vi "PH_Stepmotor_BaseClass.update Axes Config GUI.vi"(0 "VI in":refnum<vi>, 5 "error in (no error)":errorcluster) -> (14 "VI out":refnum<vi>, 19 "error out":errorcluster)   [LabVIEW 2014, in "PH_Stepmotor_BaseClass.lvlib"]
doc: "This VI is forseen to set Attributes to the related GUI element."
uses:
  PH_Stepmotor_BaseClass.lvlib
  PH_Stepmotor_BaseClass.Axis Settings.ctl
  PH_Stepmotor_BaseClass.Motor Type.ctl
  PH_Stepmotor_BaseClass.Axis Information.ctl
  PH_Stepmotor_BaseClass.Axis Activity.ctl
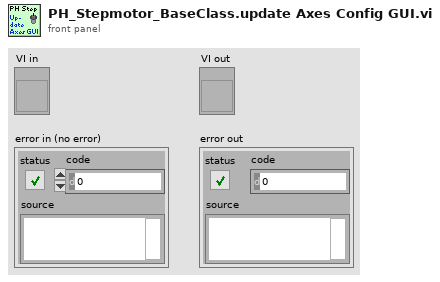
[diagram p1: front panel]
types:
  T1 = typedef "PH_Stepmotor_BaseClass.lvlib/PH_Stepmotor_BaseClass.i attribute.ctl" = cluster{"Device Error":errorcluster, "Axes PSDB Thread":cluster{"Ref":refnum<vi>, "Q-Ref":refnum<queue>, "Data Status":T2}, "Axes":T3[], "Axes PSDB Infos":cluster{"GUI Name":string, "PSDB Instance ID":i32, "PSDB Status Service ID":i32, "Axis":i32, "Class":string}[], "GUI Refs":T8}
  T2 = typedef "PH_PSDBWriter.lvlib/PH_PSDBWriter.Data Status.ctl" = i16
  T3 = typedef "PH_Stepmotor_BaseClass.lvlib/PH_Stepmotor_BaseClass.Axis Attributes.ctl" = cluster{"Settings":T4, "Endswitch?":bool, "DIM Service IDs":T6, "Activity":T7, "Configured?":bool, "Position":cluster{"Current":i32, "Target":i32}, "Position to set":cluster{"New?":bool, "Wanted":i32}, "Stop?":bool, "Reset?":bool, "Move?":bool, "Nothing connected?":bool}
  T4 = typedef "PH_Stepmotor_BaseClass.lvlib/PH_Stepmotor_BaseClass.Axis Settings.ctl" = cluster{"Sign change":bool, "Width":dbl, "Calibration":dbl, "Unit":string, "Motor Type":T5, "Unit Width":string, "Unit CF":string}
  T5 = typedef "PH_Stepmotor_BaseClass.lvlib/PH_Stepmotor_BaseClass.Motor Type.ctl" = enum16{"Unspecific", "OWIS 49.120.2633", "OWIS 49.060.1033", "OWIS 43.040.2558", "Diamond Motion 2200 series", "OWIS 49.120.266B.MV6", "Calorimeter", "Linear Stage 1", "MICOS VT-80", "MICOS VT-80 S", "Standa Rotstage nt0.95A", "PUF RA 320.200", "PUF RA 800.200", "PUF RA 800.400", "PUF RA 400.50", "1324.nn.800.50", "1324.n9c.800.50", "1324.nn.320.200", "1324.nn.400.200", "1324.nn.800.200", "1324.nn.400.50", "1324.8c9c.800.50", "1324.8c9c.400.200"}
  T6 = typedef "PH_Stepmotor_BaseClass.lvlib/PH_Stepmotor_BaseClass.Axis DIM Service IDs.ctl" = cluster{"Settings":i32, "Information":i32}
  T7 = typedef "PH_Stepmotor_BaseClass.lvlib/PH_Stepmotor_BaseClass.Axis Activity.ctl" = enum16{"No Information", "stopped", "running", "Failure", "Alarm", "stopped at backward ES", "stopped at foreward ES"}
  T8 = typedef "PH_Stepmotor_BaseClass.lvlib/PH_Stepmotor_BaseClass.GUI Refs.ctl" = cluster{"Axes Configuration":refnum<vi>, "Device Error":refnum<vi>, "Axes PSDB Infos":refnum<vi>}
  T9 = typedef "PH_Stepmotor_BaseClass.lvlib/PH_Stepmotor_BaseClass.Axis Information.ctl" = cluster{"Scaled Position":dbl, "Activity":T7}
  T10 = cluster{"Settings":T4, "Axis Information":T9, "Position":i32}
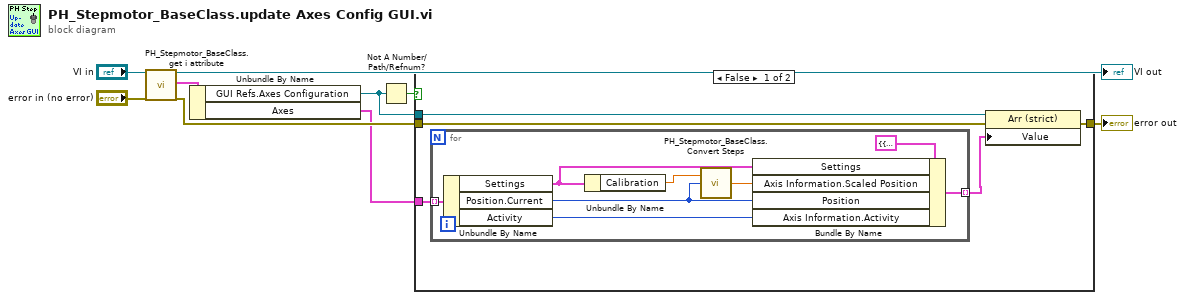
[diagram p0: block diagram]
diagram:
  n1 = call "PH_Stepmotor_BaseClass.get i attribute.vi"("i ref in"="VI in", "error in (no error)"="error in (no error)") -> ("i ref out"=→"VI out":refnum<vi>, "i attribute"=w4:T1, "error out"=w7:errorcluster)  [unwired: 15 in]
  n2 = Unbundle By Name(w4) -> ("GUI Refs.Axes Configuration"=w2:refnum<vi>, "Axes"=w1:T3[])
  n3 = Not A Number/Path/Refnum?(number/path/refnum=w2) -> (NaN/Path/Refnum?=w3:bool)
  n4 = case shown="False" w3 {
    tunnel: w7 -> [w14 w23]
    tunnel: [w13 w23] -> w5
    tunnel: w2 -> [w12 _]
    tunnel: w1 -> [w11 _]
    frame False {
      n5 = for {
        tunnel: [w22] -> w10 mode=indexing
        tunnel: w11 -> [w21] mode=indexing
        n6 = Unbundle By Name(w21) -> ("Settings"=w18:T4, "Position.Current"=w20:i32, "Activity"=w16:T7)
        n7 = Unbundle By Name(w18) -> ("Calibration"=w17:dbl)
        n8 = call "PH_Stepmotor_BaseClass.Convert Steps.vi"("Postion (steps)"=w20, "Calibration Factor"=w17) -> ("Scaled Position"=w19:dbl)
        n9 = Bundle By Name(cluster=T10 {"Settings"={"Sign change"=FALSE, "Width"=0.0, "Calibration"=0.0, "Unit"="", "Motor Type"=enum."Unspecific", "Unit Width"="", "Unit CF"=""}, "Axis Information"={"Scaled Position"=0.0, "Activity"=enum."No Information"}, "Position"=0} ("BaseClass Axis Configuration"), "Settings"=w18, "Axis Information.Scaled Position"=w19, "Position"=w20, "Axis Information.Activity"=w16) -> (w22:T10)
      }
      n10 = property class="Arr (strict)"(reference=w12, error in=w14, "Value"=w10) -> (error out=w13:errorcluster)  [unwired: 1 out]
    }
    frame True {
    }
  }
  "error out" <- w5
